vi "FreqSegments.vi"(0 "VISA resource name":refnum<visa-resource-name>, 1 "FrequenciesIn":dbl[](array[numeric]), 2 "Power":dbl, 3 "error in (no error)":errorcluster, 4 "IFBW":dbl) -> (5 "VISA resource name out":refnum<visa-resource-name>, 6 "FrequenciesOut":dbl[](array[numeric]), 7 "error out":errorcluster)   [LabVIEW 2015]
uses:
  <instrlib>/Rohde&Schwarz Vector Network Analyzer/Rohde&Schwarz Vector Network Analyzer.lvlib
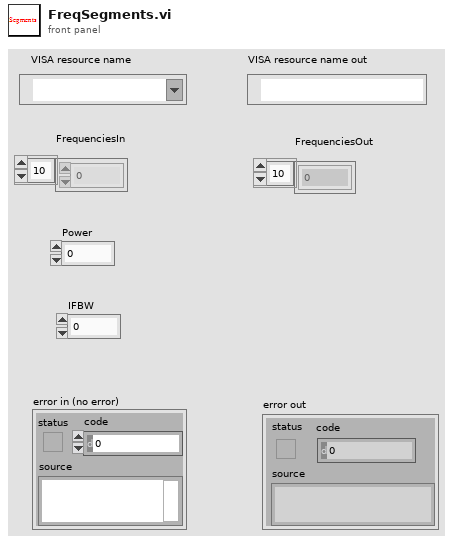
[diagram p1: front panel]
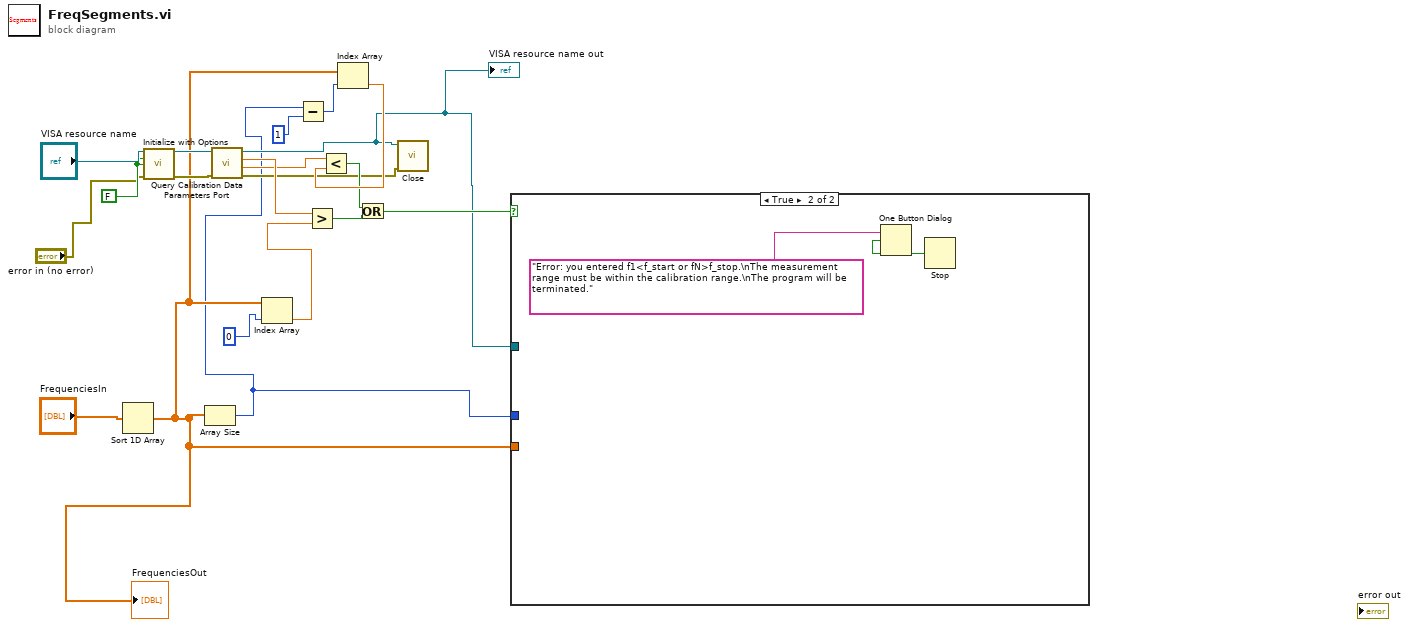
[diagram p0: block diagram]
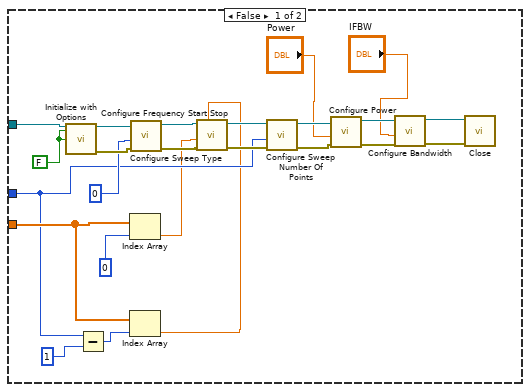
[diagram p2: hidden frame]
diagram:
  w18 = FALSE
  n1 = Sort 1D Array(array="FrequenciesIn") -> (sorted array=w2:dbl[])
  "FrequenciesOut" <- w2
  n2 = call <instrlib>:"Initialize with Options.vi"("VISA resource name"="VISA resource name", "ID Query (T: Check)"=w18, "Reset (T: Reset)"=w18, "error in (no error)"="error in (no error)") -> ("VISA resource name out"=w17:refnum<visa-resource-name>, "error out"=w16:errorcluster)  [unwired: 10 in]
  n3 = Array Size(array=w2) -> (size(s)=w1:i32)
  n4 = call <instrlib>:"Query Calibration Data Parameters Port.vi"("error in (no error)"=w16, "VISA resource name"=w17) -> ("error out"=w4:errorcluster, "Frequency Stop"=w10:dbl, "Frequency Start"=w13:dbl, "VISA resource name out"=w3:refnum<visa-resource-name>)  [unwired: 3 in, 3 out]
  "VISA resource name out" <- w3
  n5 = Index Array(array=w2, index=0) -> (element=w12:dbl)
  n6 = Subtract(x=w1, y=1) -> (x-y=w8:i32)
  n7 = Greater?(x=w13, y=w12) -> (0:w11:bool)
  n8 = Index Array(array=w2, index=w8) -> (element=w7:dbl)
  n9 = Less?(x=w10, y=w7) -> (x < y?=w6:bool)
  n10 = Or(x=w6, y=w11) -> (x .or. y?=w5:bool)
  n11 = call <instrlib>:"Close.vi"("error in (no error)"=w4, "VISA resource name"=w3) -> ()  [unwired: 9 in, 1 out]
  n12 = case shown="True" w5 {
    tunnel: w3 -> [w42 _]
    tunnel: w2 -> [w26 _]
    tunnel: w1 -> [w24 _]
    frame False {
      w44 = FALSE
      n13 = call <instrlib>:"Initialize with Options.vi"("VISA resource name"=w42, "ID Query (T: Check)"=w44, "Reset (T: Reset)"=w44) -> ("VISA resource name out"=w41:refnum<visa-resource-name>, "error out"=w40:errorcluster)  [unwired: 11 in]
      n14 = Subtract(x=w24, y=1) -> (x-y=w25:i32)
      n15 = Index Array(array=w26, index=0) -> (element=w22:dbl)
      n16 = Index Array(array=w26, index=w25) -> (element=w21:dbl)
      n17 = call <instrlib>:"Configure Sweep Type.vi"("error in (no error)"=w40, "Sweep Type (Power)"=0, "VISA resource name"=w41) -> ("error out"=w35:errorcluster, "VISA resource name out"=w34:refnum<visa-resource-name>)  [unwired: 7 in]
      n18 = call <instrlib>:"Configure Frequency Start Stop.vi"("Stop Frequency (4.0e9)"=w21, "error in (no error)"=w35, "Start Frequency (300.0e3)"=w22, "VISA resource name"=w34) -> ("error out"=w33:errorcluster, "VISA resource name out"=w32:refnum<visa-resource-name>)  [unwired: 6 in]
      n19 = call <instrlib>:"Configure Sweep Number Of Points.vi"("error in (no error)"=w33, "Number Of Points (201)"=w24, "VISA resource name"=w32) -> ("error out"=w36:errorcluster, "VISA resource name out"=w39:refnum<visa-resource-name>)  [unwired: 7 in]
      n20 = call <instrlib>:"Configure Power.vi"("error in (no error)"=w36, "Power (-10.0)"="Power", "VISA resource name"=w39) -> ("error out"=w38:errorcluster, "VISA resource name out"=w37:refnum<visa-resource-name>)  [unwired: 7 in]
      n21 = call <instrlib>:"Configure Bandwidth.vi"("error in (no error)"=w38, "Bandwidth (10.0e3)"="IFBW", "VISA resource name"=w37) -> ("error out"=w27:errorcluster, "VISA resource name out"=w28:refnum<visa-resource-name>)  [unwired: 7 in]
      n22 = call <instrlib>:"Close.vi"("error in (no error)"=w27, "VISA resource name"=w28) -> ()  [unwired: 9 in, 1 out]
    }
    frame True {
      n23 = One Button Dialog(message="Error: you entered f1<f_start or fN>f_stop.\nThe measurement range must be within the calibration range.\nThe program will be terminated.") -> (true=w46:bool)  [unwired: 1 in]
      n24 = Stop(stop? (T)=w46) -> ()
    }
  }
